vi "Generate Status-API Mapping mermaid.vi"(8 "Error in":errorcluster caption="Error in (no error)") -> (0 "Error out":errorcluster, 2 "Array":T2(array[cluster]), 3 "String":string)   [LabVIEW 2020]
uses:
  <userlib>/_NEVSTOP/Communicable State Machine(CSM)/Communicable State Machine.lvlib
  <userlib>/_NEVSTOP/Communicable State Machine(CSM)/AdvanceAPI/CSM - Broadcast Message Type.ctl
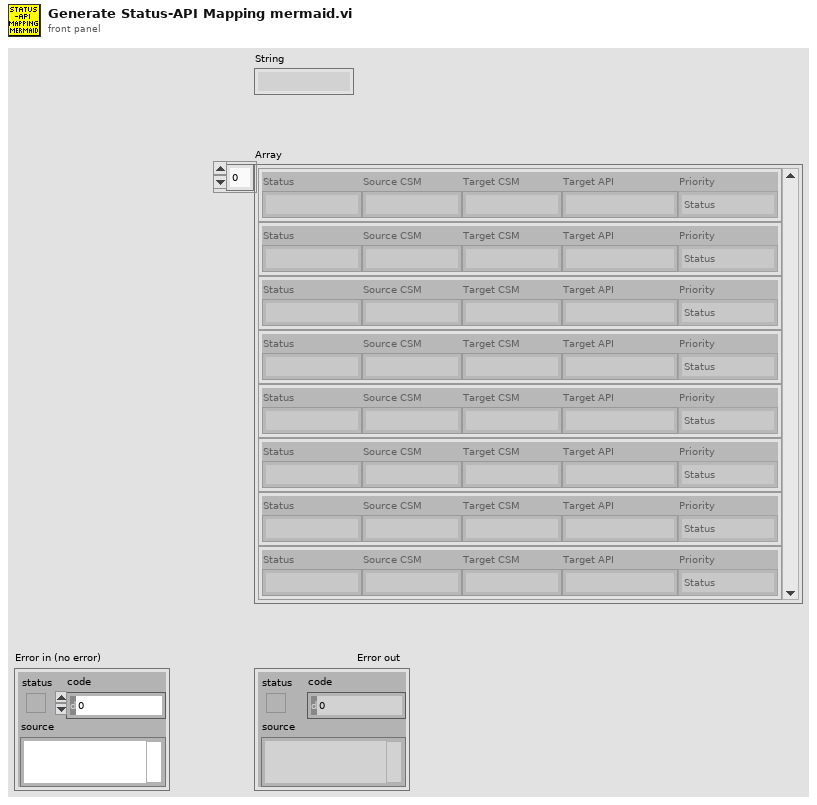
[diagram p1: front panel]
types:
  T1 = typedef "Communicable State Machine.lvlib/CSM - Broadcast Message Type.ctl" = enum16{"Status", "Interrupt(High)"}
  T2 = cluster{"Status":string, "Source CSM":string, "Target CSM":string, "Target API":string, "Priority":T1}[]
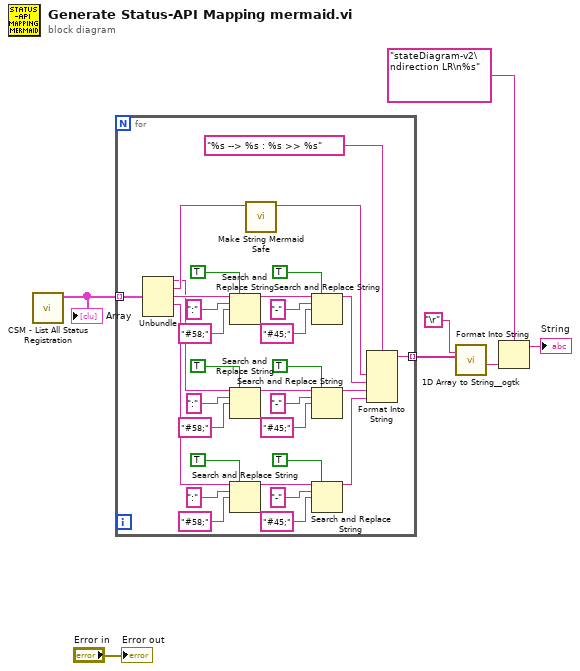
[diagram p0: block diagram]
diagram:
  n1 = call <userlib>:"CSM - List All Status Registration.vi"() -> ("Array"=w5:T2)  [unwired: 10 in, 1 out]
  "Array" <- w5
  n2 = for {
    tunnel: w5 -> [w39] mode=indexing
    tunnel: [w37] -> w4 mode=indexing
    n3 = Unbundle(w39) -> ("Status"=w9:string, "Source CSM"=w18:string, "Target CSM"=w35:string, "Target API"=w29:string)  [unwired: 1 out]
    n4 = Search and Replace String(replace all?=TRUE ("replace all? (F)"), input string=w35, search string=":", replace string="#58;" ("search string")) -> (result string=w25:string)  [unwired: 4 in, 3 out]
    n5 = Search and Replace String(replace all?=TRUE ("replace all? (F)"), input string=w9, search string=":", replace string="#58;" ("search string")) -> (result string=w10:string)  [unwired: 4 in, 3 out]
    n6 = Search and Replace String(replace all?=TRUE ("replace all? (F)"), input string=w29, search string=":", replace string="#58;" ("search string")) -> (result string=w20:string)  [unwired: 4 in, 3 out]
    n7 = call "Make String Mermaid Safe.vi"("Source CSM"=w18) -> ("result string"=w17:string)  [unwired: 10 in]
    n8 = Search and Replace String(replace all?=TRUE ("replace all? (F)"), input string=w25, search string="-", replace string="#45;" ("search string")) -> (result string=w24:string)  [unwired: 4 in, 3 out]
    n9 = Search and Replace String(replace all?=TRUE ("replace all? (F)"), input string=w10, search string="-", replace string="#45;" ("search string")) -> (result string=w8:string)  [unwired: 4 in, 3 out]
    n10 = Search and Replace String(replace all?=TRUE ("replace all? (F)"), input string=w20, search string="-", replace string="#45;" ("search string")) -> (result string=w19:string)  [unwired: 4 in, 3 out]
    n11 = Format Into String(format string="%s --> %s : %s >> %s", w17, w24, w8, w19) -> (resulting string=w37:string)  [unwired: 2 in, 1 out]
  }
  n12 = call <userlib>:"1D Array to String__ogtk.vi"("delimiter (Tab)"="\r", "Array of Strings"=w4) -> ("delimited string"=w3:string)  [unwired: 9 in]
  n13 = Format Into String(format string="stateDiagram-v2\ndirection LR\n%s", w3) -> (resulting string=→"String":string)  [unwired: 2 in, 1 out]
  "Error out" <- "Error in"
